vi "prepare buffer array without mem init.vi"(7 "shots# per page":i32, 8 "error in (no error)":errorcluster, 9 "shot H":i32, 10 "page W":i32, 11 "buffer page #":i32) -> (0 "error out":errorcluster, 2 "Image array":T1[](array[typedef]), 3 "ptr array":u64[](array[numeric]))   [LabVIEW 2021, in "Camera.lvlib" / "Camera.lvclass"]
uses:
  Camera.lvclass
  <vilib>/vision/Image Controls.llb/IMAQ Image.ctl
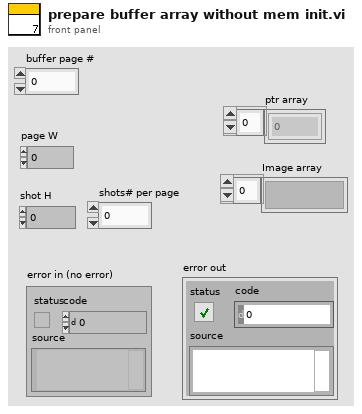
[diagram p1: front panel]
types:
  T1 = typedef "IMAQ Image.ctl" = refnum<image>
  T2 = enum32{"Map Pixel Pointer", "Unmap Pixel Pointer", "Get Pixels Infos"}
  T3 = typedef "Image Type" = u32
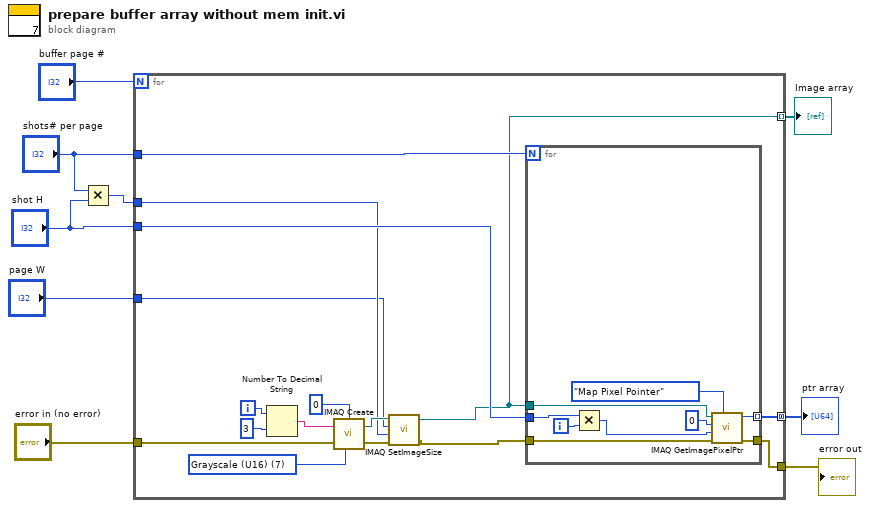
[diagram p0: block diagram]
diagram:
  n1 = Multiply(x="shots# per page", y="shot H") -> (x*y=w1:i32)
  n2 = for {
    N: "buffer page #" -> [_]
    tunnel: "page W" -> [w12]
    tunnel: w1 -> [w13]
    tunnel: "error in (no error)" -> [w18]
    tunnel: "shots# per page" -> [w17]
    tunnel: "shot H" -> [w16]
    tunnel: [w15] -> w7 mode=concatenating
    tunnel: [w14] -> w6
    tunnel: [w11] -> w3 mode=indexing
    i -> [w24]
    w22 = T3 7 items=["Grayscale (U8)", "Grayscale (I16)", "Grayscale (SGL)", "Complex (CSG)", "RGB (U32)", "HSL (U32)", "RGB (U64)", "Grayscale (U16)"] ("Image Type")
    n3 = Number To Decimal String(number=w24, width (-)=i16 3) -> (decimal integer string=w21:string)
    n4 = call "IMAQ Create"("Border Size"=0, "Image Name"=w21, "Image Type"=w22, "error in (no error)"=w18) -> ("New Image"=w20:T1, "error out"=w19:errorcluster)  [unwired: 1 in]
    n5 = call "IMAQ SetImageSize"("error in (no error)"=w19, "Y Resolution"=w13, "X Resolution"=w12, "Image"=w20) -> ("error out"=w10:errorcluster, "Image Out"=w11:T1)  [unwired: 1 in]
    n6 = for {
      N: w17 -> [_]
      tunnel: w16 -> [w33]
      tunnel: w11 -> [w29]
      tunnel: w10 -> [w30]
      tunnel: [w27] -> w15 mode=indexing
      tunnel: [w26] -> w14
      i -> [w32]
      n7 = Multiply(x=w33, y=w32) -> (x*y=w31:i32)
      n8 = call "IMAQ GetImagePixelPtr"("Function"=T2."Map Pixel Pointer", "error in (no error)"=w30, "Y Coordinate"=w31, "X Coordinate"=0, "Image"=w29) -> ("error out"=w26:errorcluster, "Pixel Pointer out"=w27:u64)  [unwired: 1 in, 4 out]
    }
  }
  "ptr array" <- w7
  "error out" <- w6
  "Image array" <- w3
